vi "Generate HTTP header.vi"(4 "error out":errorcluster, 5 "Path":string, 6 "Port":i32, 7 "Server":string) -> (0 "error IO":errorcluster, 3 "HTTP Header":string)   [LabVIEW 2020, in "Feed.lvclass"]
uses:
  <vilib>/NI_RSS/Feed/Feed.lvclass
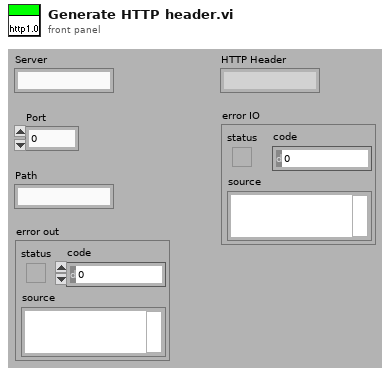
[diagram p1: front panel]
types:
  T1 = enum32{"invalid OS target", "Mac OS", "Windows 3.1", "Windows 95/NT", "Solaris 1", "Solaris 2", "HP-UX", "PowerMAX", "Linux", "Irix", "Rhapsody", "BeOS", "AIX", "OSF1", "VxWorks", "PharLap", "Carbon", "RTX", "Windows x64", "Linux x64", "Mac OS X x64"}
  T2 = enum32{"invalid CPU target", "Motorola 68K", "PowerPC", "Intel x86", "SPARC", "PA-RISC", "MIPS", "Alpha", "ARM", "AMD/Intel x64"}
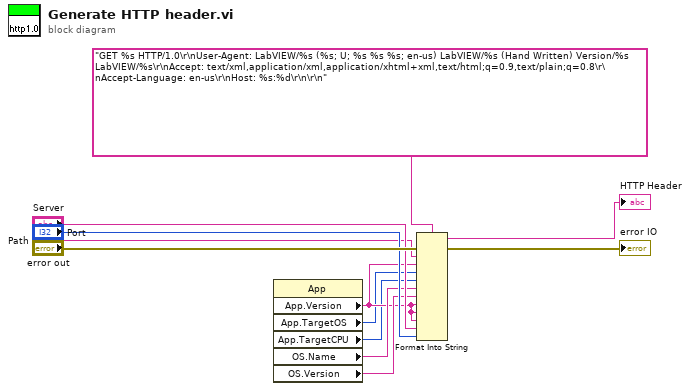
[diagram p0: block diagram]
diagram:
  n1 = property class="App"() -> ("App.Version"=w5:string, "App.TargetOS"=w4:T1, "App.TargetCPU"=w2:T2, "OS.Name"=w8:string, "OS.Version"=w7:string)  [unwired: 2 in, 2 out]
  n2 = Format Into String(format string="GET %s HTTP/1.0\r\nUser-Agent: LabVIEW/%s (%s; U; %s %s %s; en-us) LabVIEW/%s (Hand Written) Version/%s LabVIEW/%s\r\nAccept: text/xml,application/xml,application/xhtml+xml,text/html;q=0.9,text/plain;q=0.8\r\nAccept-Language: en-us\r\nHost: %s:%d\r\n\r\n", error in="error out", "Path", w5, w4, w2, w8, w7, w5, w5, w5, "Server", "Port") -> (resulting string=→"HTTP Header":string, error out=→"error IO":errorcluster)  [unwired: 1 in]
